vi "getRegisters.vi"(0 "WaveformAddressSpace in":refnum<class "WaveformAddressSpace.lvclass">) -> (4 "WaveformAddressSpace out":refnum<class "WaveformAddressSpace.lvclass">, 6 "Registers":T1={"oclk_freq"="oclk freq", "data_rate"="data rate", "oclk_div"="oclk div", "oclk_mult"="oclk mult", "AcquisitionType"="Acquisition Type", "SamplesPerChan"="Samps per Chan", "NumberOfChannels"="Number of Channels", "stop"="Register", "FIFO"="DataSGL", "FirstRead"="FirstRead", "ErrorCode"="ErrorCode", "ChannelCount"="ChannelCount", "Finished"="Finished", "DMA_FIFO_Full"="DMA FIFO Full", "ModuleUnderflow"="Module Underflow", "ConfigReadyRead"="Register", "ConfigReadyWrite"="Register", "SynchStartRead"="Register", "SynchStartWrite"="Register", "UnderflowCount"=""})   [LabVIEW 2015]
uses:
  WaveformAddressSpace.lvclass
  Registers.ctl
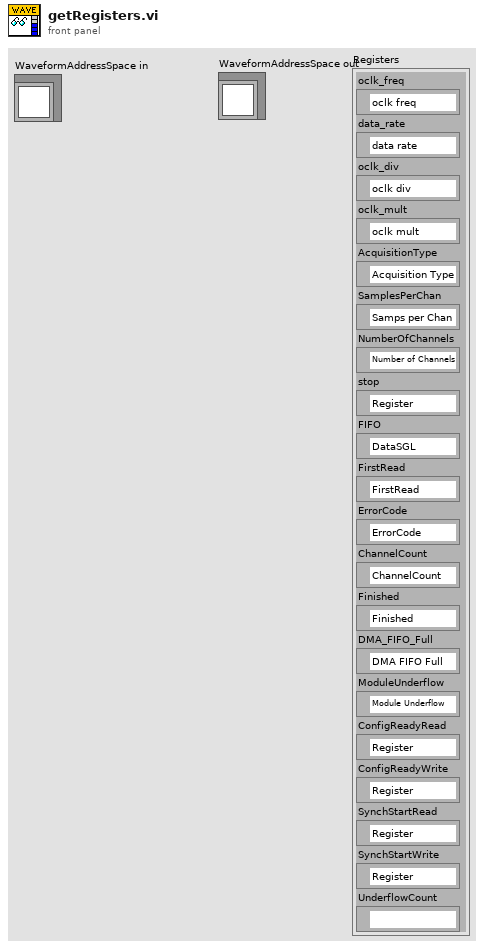
[diagram p1: front panel]
types:
  T1 = typedef "WaveformAddressSpace.lvclass/Registers.ctl" = cluster{"oclk_freq":refnum<k21>, "data_rate":refnum<k21>, "oclk_div":refnum<k21>, "oclk_mult":refnum<k21>, "AcquisitionType":refnum<k21>, "SamplesPerChan":refnum<k21>, "NumberOfChannels":refnum<k21>, "stop":refnum<k21>, "FIFO":refnum<k21>, "FirstRead":refnum<k21>, "ErrorCode":refnum<k21>, "ChannelCount":refnum<k21>, "Finished":refnum<k21>, "DMA_FIFO_Full":refnum<k21>, "ModuleUnderflow":refnum<k21>, "ConfigReadyRead":refnum<k21>, "ConfigReadyWrite":refnum<k21>, "SynchStartRead":refnum<k21>, "SynchStartWrite":refnum<k21>, "UnderflowCount":refnum<k21>}
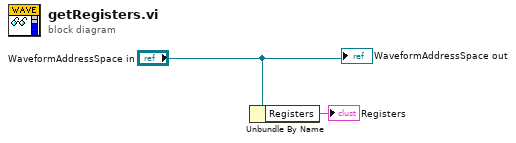
[diagram p0: block diagram]
diagram:
  n1 = Unbundle By Name("WaveformAddressSpace in") -> ("Registers"=→"Registers")
  "WaveformAddressSpace out" <- "WaveformAddressSpace in"
